vi "Control Panel Initialization Message.vi"(8 "error in (no error)":errorcluster, 10 "Resource":variant, 11 "Generic Optimizer in":refnum<class "Generic Optimizer.lvclass">) -> (0 "error out":errorcluster, 2 "Message":T1, 3 "Generic Optimizer out":refnum<class "Generic Optimizer.lvclass">)   [LabVIEW 2020, in "Generic Optimizer.lvclass"]
doc: "Method to generate the initial message to send to a Controller's Control Panel."
uses:
  Generic Optimizer.lvclass
  <userlib>/Dynamic Reentrant/Type Defs/Message.ctl
  <userlib>/Dynamic Reentrant/Dynamic Reentrant.lvlib
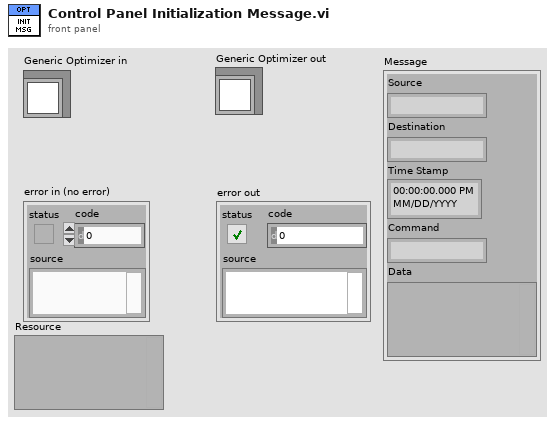
[diagram p1: front panel]
types:
  T1 = typedef "Dynamic Reentrant.lvlib/Message.ctl" = cluster{"Source":string, "Destination":string, "Time Stamp":timestamp, "Command":string, "Data":variant}
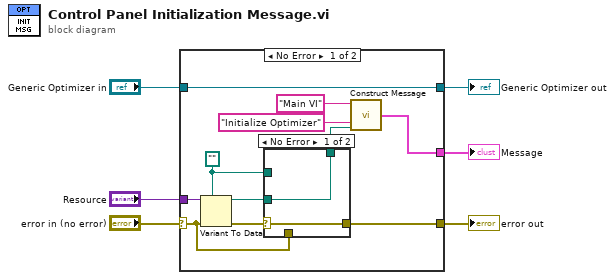
[diagram p0: block diagram]
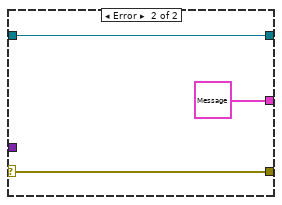
[diagram p3: hidden frame]
diagram:
  n1 = case shown="No Error" "error in (no error)" {
    selector: "error in (no error)" -> [w11 w23]
    tunnel: [w10 w23] -> w5
    tunnel: [w17 w24] -> w3
    tunnel: "Generic Optimizer in" -> [w17 w24]
    tunnel: [w16 T1 {"Source"="", "Destination"="", "Time Stamp"=timestamp(0 s since 1904-01-01), "Command"="", "Data"=variant} ("Message")] -> w2
    tunnel: "Resource" -> [w13 _]
    frame No Error {
      w9 = path ""
      n2 = Variant To Data(error in=w11, type=w9, Variant=w13) -> (data=w8:path, error out=w12:errorcluster)
      n3 = case shown="No Error" w12 {
        selector: w12 -> [w18 _]
        tunnel: w9 -> [_ w21]
        tunnel: w8 -> [w19 _]
        tunnel: [w19 w21] -> w7
        tunnel: [w18 w20] -> w10
        tunnel: w11 -> [_ w20]
        frame No Error {
        }
        frame Error {
        }
      }
      n4 = call <userlib>:"Construct Message.vi"("Data"=w7, "Command"="Initialize Optimizer", "Source"="Main VI") -> ("output cluster"=w16:T1)  [unwired: 3 in]
    }
    frame Error {
    }
  }
  "Generic Optimizer out" <- w3
  "error out" <- w5
  "Message" <- w2
